vi "AtDome_salEvent_emergencyStop.vi"(8 "error in (no error)":errorcluster) -> (0 "error out":errorcluster, 3 "function return":i32)   [LabVIEW 2016, in "SALLV_AtDome.lvlib"]
doc: "int AtDome_shm_salEvent_emergencyStopLV();"
uses:
  SALLV_AtDome.lvlib
  SALLV_AtDome.so
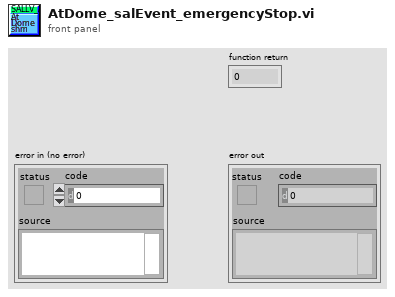
[diagram p1: front panel]
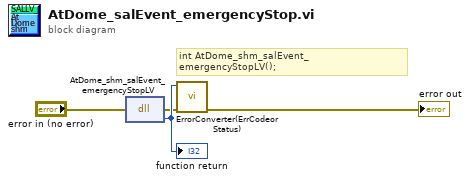
[diagram p0: block diagram]
diagram:
  # "int AtDome_shm_salEvent_emergencyStopLV();"
  n1 = dll-call lib="home/andres/Desktop/SAL_AtDome/SALLV_AtDome.*" fn="AtDome_shm_salEvent_emergencyStopLV"(error in="error in (no error)") -> (error out=w2:errorcluster, w4:i32)  [unwired: 2 in, 1 out]
  "function return" <- w4
  n2 = call "ErrorConverter(ErrCodeorStatus).vi"("error in (no error)"=w2, "error code"=w4) -> ("error out"=→"error out":errorcluster)  [unwired: 9 in]
